vi "Set value by string.vi"(8 "error in (no error)":errorcluster, 10 "Value":string, 11 "Column in":refnum<class "Column Parent.lvclass">) -> (0 "error out":errorcluster, 3 "Column out":refnum<class "Column Parent.lvclass">)   [LabVIEW 2020, in "Basic Columns.lvlib" / "Column Parent.lvclass"]
uses:
  Column Parent.lvclass
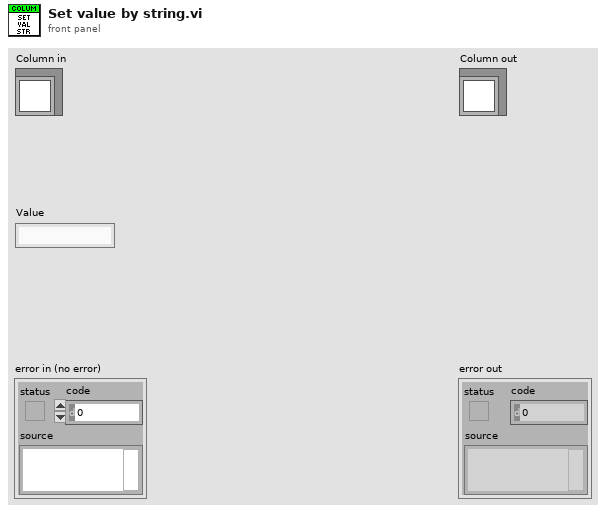
[diagram p1: front panel]
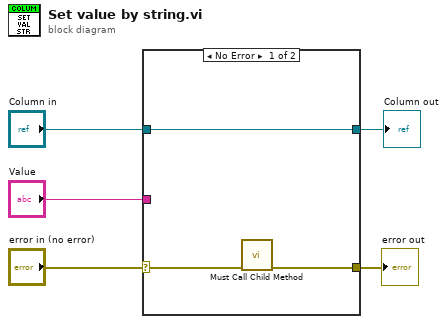
[diagram p0: block diagram]
diagram:
  n1 = case shown="No Error" "error in (no error)" {
    selector: "error in (no error)" -> [w7 w9]
    tunnel: [w6 w9] -> w4
    tunnel: "Column in" -> [w8 w10]
    tunnel: [w8 w10] -> w2
    tunnel: "Value" -> [_ _]
    frame No Error {
      n2 = call "Must Call Child Method.vi"("error in"=w7) -> ("error out"=w6:errorcluster)  [unwired: 10 in]
    }
    frame Error {
    }
  }
  "error out" <- w4
  "Column out" <- w2
